vi "Log Motors.vi"(4 "Target Torque Right":i16(knob) scale=1000.0..-1000.0, 5 "Target Torque Left":i16(knob) scale=-1000.0..1000.0, 6 "Right Motor Status":T2, 7 "Left Motor Status":T2, 8 "\"Pedals\" Status":T1 {"Acceleration pedal" scale=0.0..100.0 scale format="%#_6f%%"; "Break pedal" scale=0.0..100.0 scale format="%#_6f%%"}, 9 "Log File Cluster":T3) -> ()   [LabVIEW 2016]
uses:
  Log File Cluster.ctl
  RT/Pedals Status.ctl
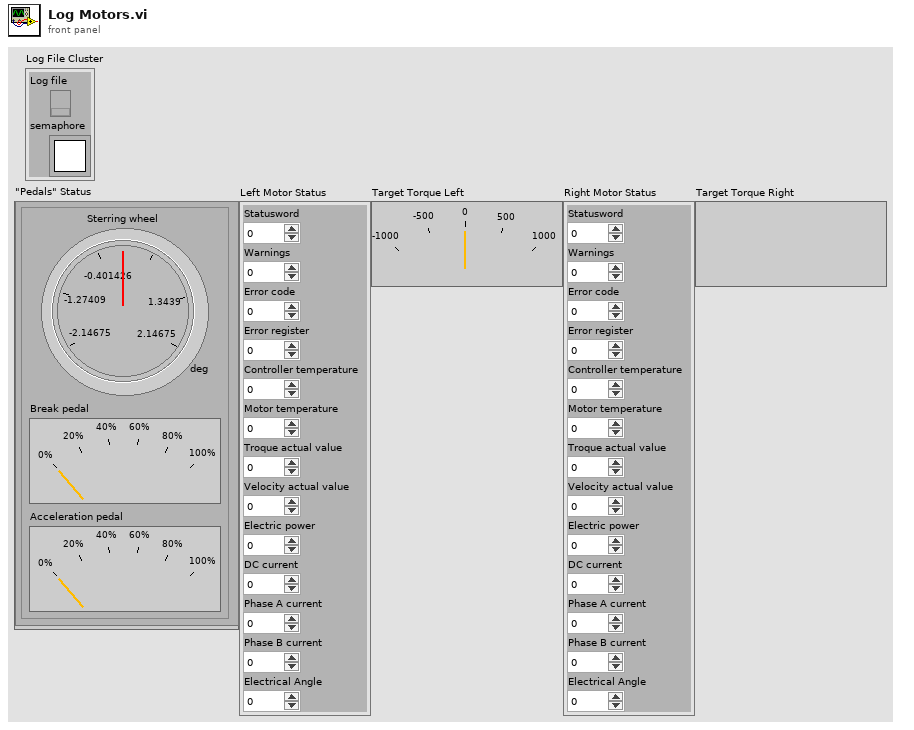
[diagram p1: front panel]
types:
  T1 = typedef "Pedals Status.ctl" = cluster{"Acceleration pedal":dbl, "Break pedal":dbl, "Sterring wheel":dbl[unit]}
  T2 = cluster{"Statusword":u16, "Warnings":u16, "Error code":u16, "Error register":u8, "Controller temperature":u8, "Motor temperature":u8, "Troque actual value":i16, "Velocity actual value":i32, "Electric power":u32, "DC current":u32, "Phase A current":u16, "Phase B current":u16, "Electrical Angle":u16}
  T3 = typedef "Log File Cluster.ctl" = cluster{"Log file":refnum<k34>, "semaphore":T4}
  T4 = typedef "Semaphore RefNum" = refnum<k1>
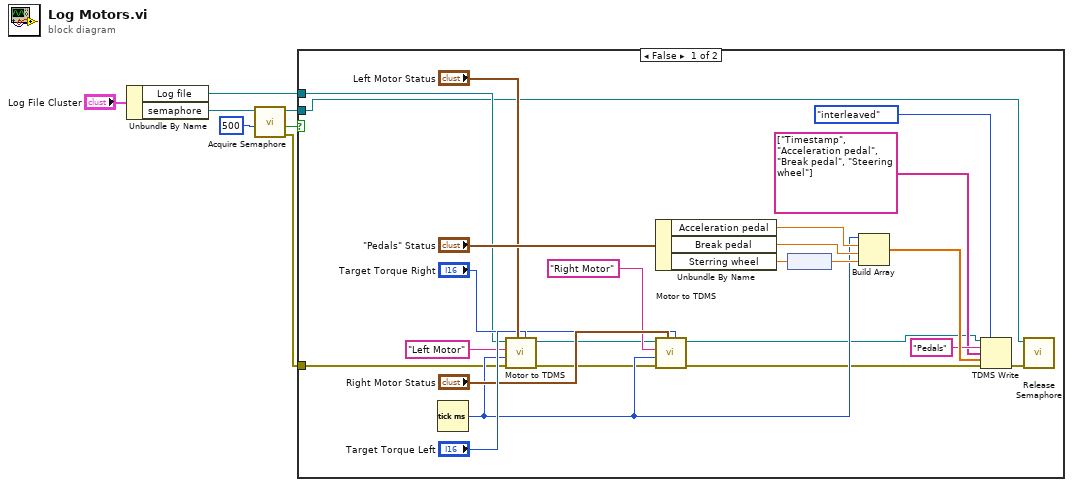
[diagram p0: block diagram]
diagram:
  n1 = Unbundle By Name("Log File Cluster") -> ("Log file"=w6:refnum<k34>, "semaphore"=w4:T4)
  n2 = call <vilib>:"Acquire Semaphore.vi"("ms timeout (-1)"=500, "semaphore"=w4) -> ("error out"=w5:errorcluster, "timed out"=w1:bool, "semaphore out"=w2:T4)  [unwired: 3 in]
  n3 = case shown="False" w1 {
    tunnel: w6 -> [w18 _]
    tunnel: w5 -> [w14 _]
    tunnel: w2 -> [w13 _]
    frame False {
      n4 = Tick Count (ms)() -> (millisecond timer value=w15:u32)
      n5 = call "Motor to TDMS.vi"("Target Torque"="Target Torque Left", "Motor Status"="Left Motor Status", "error in (no error)"=w14, "Timestamp"=w15, "group name in (Untitled)"="Left Motor", "tdms file"=w18) -> ("error out"=w10:errorcluster, "tdms file out"=w11:refnum<k34>)  [unwired: 3 in, 1 out]
      n6 = Unbundle By Name("\"Pedals\" Status") -> ("Acceleration pedal"=w30:dbl, "Break pedal"=w29:dbl, "Sterring wheel"=w28:dbl[unit])
      n7 = call "Motor to TDMS.vi"("Target Torque"="Target Torque Right", "Motor Status"="Right Motor Status", "error in (no error)"=w10, "Timestamp"=w15, "group name in (Untitled)"="Right Motor", "tdms file"=w11) -> ("error out"=w8:errorcluster, "tdms file out"=w9:refnum<k34>)  [unwired: 3 in, 1 out]
      n8 = node(w28) -> (w27:dbl)
      n9 = Build Array(w15, w30, w29, w27) -> (w26:dbl[])
      n10 = TDMS Write(0:w9, 1:enum16{"decimated", "interleaved"}."interleaved" ("data layout (0:decimated)"), 5:"Pedals" ("group name in (Untitled)"), 7:string[] ["Timestamp", "Acceleration pedal", "Break pedal", "Steering wheel"], 9:w26, 11:w8) -> (15:w12:errorcluster)  [unwired: 3 out]
      n11 = call <vilib>:"Release Semaphore.vi"("error in (no error)"=w12, "semaphore"=w13) -> ()  [unwired: 4 in, 2 out]
    }
    frame True {
    }
  }
